vi "az_ellenseg_megtevesztese.vi"() -> ()   [LabVIEW 2018]
uses:
  <vilib>/NI/STM/TCP/TCP Connection Info.ctl
  <vilib>/NI/STM/SubVIs/MetaDataElement.ctl
  <vilib>/NI/STM/TCP/TCP Write Options.ctl
  <vilib>/NI/STM/TCP/TCP Read Options.ctl
  <vilib>/NI/STM/TCP/Write Meta Data (TCP Ref).vi
  <vilib>/NI/STM/TCP/Get Connection Reference (TCP).vi
  <vilib>/NI/STM/TCP/Write Meta Data (TCP Clst).vi
  <vilib>/NI/STM/TCP/Read Message (TCP).vi
  <vilib>/NI/STM/TCP/Write Message (TCP).vi
  <vilib>/NI/STM/NI STM.lvlib
panel:
  out "Sensor not connected":bool
  out "Connected?":bool
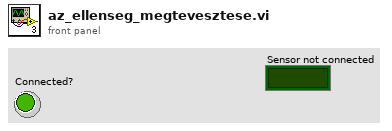
[diagram p1: front panel]
types:
  T1 = typedef "NI STM.lvlib/TCP Connection Info.ctl" = cluster{"connection ID":refnum<k5>, "meta data":T2[]}
  T2 = typedef "NI STM.lvlib/MetaDataElement.ctl" = string
  T3 = typedef "NI STM.lvlib/TCP Write Options.ctl" = cluster{"ignore timeout error":bool, "timeout ms (1000)":i32}
  T4 = typedef "NI STM.lvlib/TCP Read Options.ctl" = cluster{"ignore timeout error":bool, "timeout ms (1000)":i32}
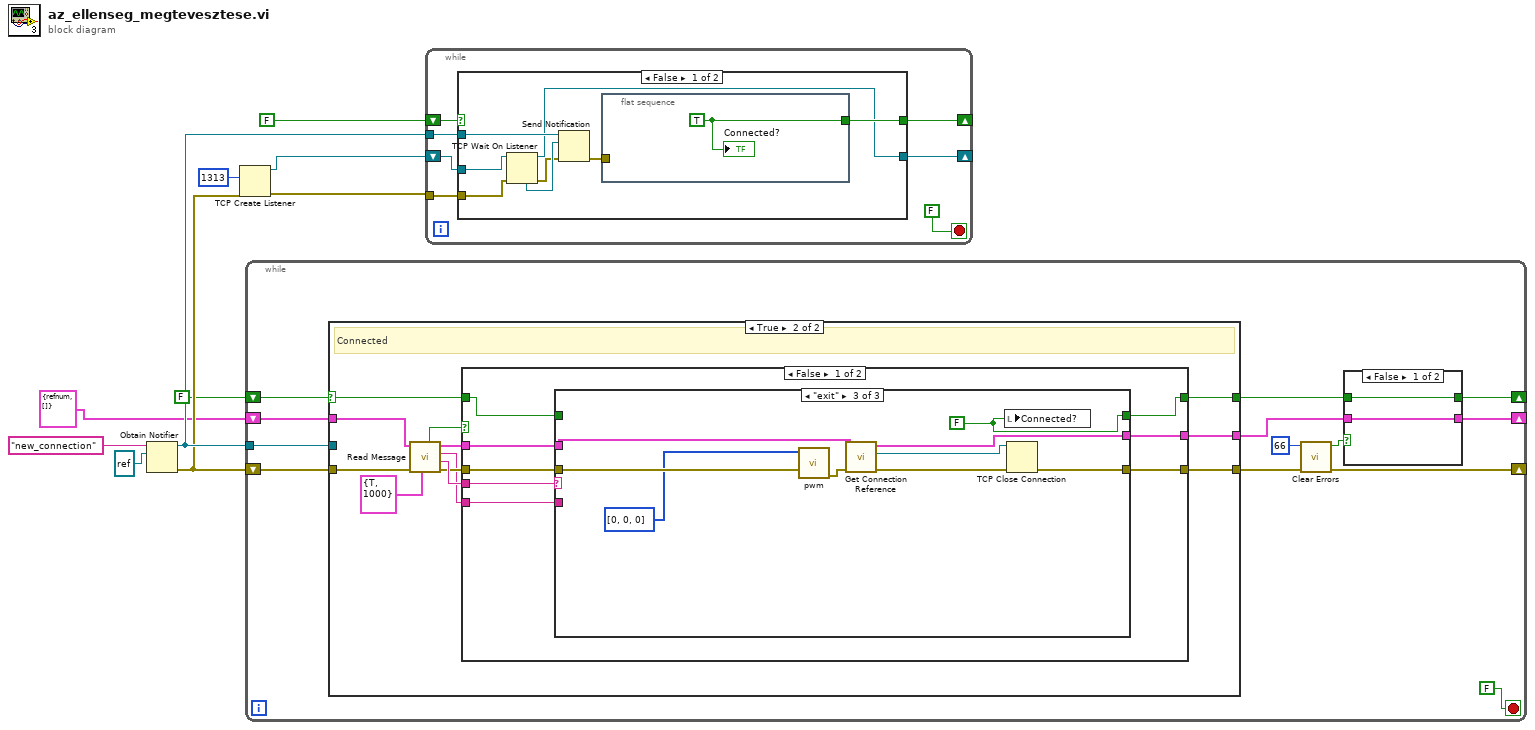
[diagram p0: block diagram]
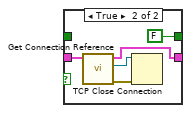
[diagram p2: hidden frame]
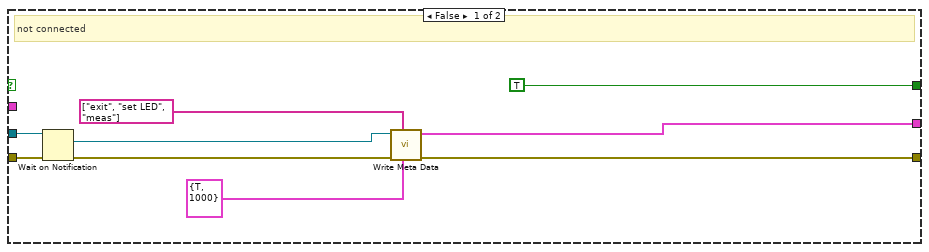
[diagram p3: hidden frame]
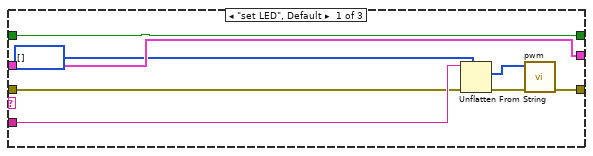
[diagram p4: hidden frame]
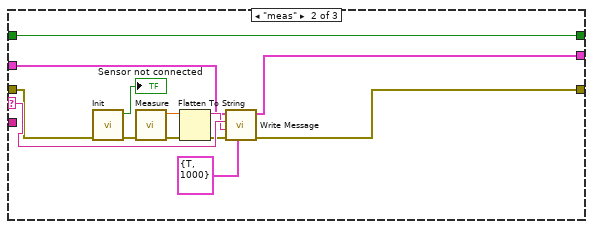
[diagram p5: hidden frame]
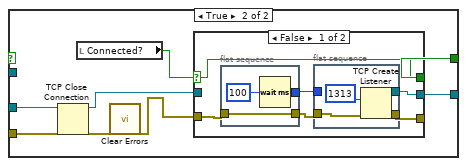
[diagram p7: hidden frame]
diagram:
  n1 = Obtain Notifier(name (unnamed)="new_connection", notification data type=refnum<k5> refnum ("connection ID")) -> (notifier out=w5:refnum<notifier>, error out=w4:errorcluster)  [unwired: 2 in, 1 out]
  n2 = TCP Create Listener(8:w4, 10:u16 1313 ("port")) -> (0:w9:errorcluster, 3:w10:refnum<k5>)  [unwired: 3 in, 1 out]
  n3 = while {
    tunnel: w5 -> [w23]
    shift-right: [w13] -> _
    shift-left: FALSE ("Connected?") -> [w21]
    shift-right: [w11] -> _
    shift-left: T1 {"connection ID"=refnum, "meta data"=[]} ("connection info out") -> [w20]
    shift-right: [w17] -> _
    shift-left: w4 -> [w18]
    stop <- FALSE stop-if-true
    n4 = case shown="True" w21 {
      selector: w21 -> [_ w41]
      tunnel: w23 -> [w39 _]
      tunnel: [TRUE w42] -> w14
      tunnel: [w36 w44] -> w12
      tunnel: w20 -> [_ w50]
      tunnel: [w32 w43] -> w19
      tunnel: w18 -> [w31 w51]
      frame False {
        # "not connected"
        n5 = Wait on Notification(notifier=w39, error in (no error)=w31) -> (notification=w37:refnum<k5>, error out=w35:errorcluster)  [unwired: 2 in, 2 out]
        n6 = call-poly <vilib>:"Write Meta Data.vi"("options"=T3 {"ignore timeout error"=TRUE, "timeout ms (1000)"=1000}, "meta data"=T2[] ["exit", "set LED", "meas"], "error in"=w35, "connection ID"=w37) -> ("error out"=w32:errorcluster, "connection info out"=w36:T1)  [unwired: 6 in]
      }
      frame True {
        # "Connected"
        n7 = call-poly <vilib>:"Read Message.vi"("options"=T4 {"ignore timeout error"=TRUE, "timeout ms (1000)"=1000}, "error in"=w51, "connection info in"=w50) -> ("error out"=w46:errorcluster, "name"=w47:T2, "data string"=w40:string, "connection info out"=w45:T1, "timed out?"=w48:bool)  [unwired: 3 in, 1 out]
        n8 = case shown="False" w48 {
          tunnel: w47 -> [w59 _]
          tunnel: w46 -> [w57 w91]
          tunnel: w45 -> [w58 w92]
          tunnel: [w56 w92] -> w44
          tunnel: [w55 w91] -> w43
          tunnel: [w54 w90] -> w42
          tunnel: w41 -> [w53 w90]
          tunnel: w40 -> [w52 _]
          frame False {
            n9 = case shown="\"exit\"" w59 {
              selector: w59 -> [_ w76 _]
              tunnel: w58 -> [w66 w73 w89]
              tunnel: w57 -> [w61 w70 w83]
              tunnel: [w66 w78 w88] -> w56
              tunnel: [w60 w79 w85] -> w55
              tunnel: [w67 w80 w84] -> w54
              tunnel: w53 -> [w67 w80 _]
              tunnel: w52 -> [w62 _ _]
              frame "set LED", Default {
                n10 = Unflatten From String(type=u8[] [], binary string=w62, error in (no error)=w61) -> (value=w64:u8[], error out=w65:errorcluster)  [unwired: 2 in, 1 out]
                n11 = call "pwm.vi"("Error In"=w65, "PWMs"=w64) -> ("Error Out"=w60:errorcluster)  [unwired: 9 in]
              }
              frame "meas" {
                n12 = call "Init.vi"("Error In"=w70) -> ("Error Out"=w69:errorcluster, "Not connected"=→"Sensor not connected":bool)  [unwired: 9 in]
                n13 = call "Measure.vi"("Error In"=w69) -> ("Error Out"=w72:errorcluster, "Luminosity"=w71:dbl)  [unwired: 9 in]
                n14 = Flatten To String(anything=w71, error in (no error)=w72) -> (data string=w74:string, error out=w75:errorcluster)  [unwired: 2 in, 1 out]
                n15 = call-poly <vilib>:"Write Message.vi"("options"=T3 {"ignore timeout error"=TRUE, "timeout ms (1000)"=1000}, "error in"=w75, "data"=w74, "name"=w76, "connection info in"=w73) -> ("error out"=w79:errorcluster, "connection info out"=w78:T1)  [unwired: 5 in]
              }
              frame "exit" {
                w84 = FALSE ("Connected?")
                n16 = call "pwm.vi"("Error In"=w83, "PWMs"=u8[] [0, 0, 0]) -> ("Error Out"=w82:errorcluster)  [unwired: 9 in]
                n17 = call-poly <vilib>:"Get Connection Reference.vi"("error in"=w82, "connection info in"=w89) -> ("error out"=w87:errorcluster, "connection ID out"=w86:refnum<k5>, "connection info out"=w88:T1)  [unwired: 7 in]
                n18 = local write "Connected?"(w84) -> ()
                n19 = TCP Close Connection(connection ID=w86, error in (no error)=w87) -> (error out=w85:errorcluster)  [unwired: 1 in, 1 out]
              }
            }
          }
          frame True {
          }
        }
      }
    }
    n20 = call <vilib>:"Clear Errors.vi"("error in (no error)"=w19, "specific error code to clear (0: all)"=66) -> ("error out"=w17:errorcluster, "specific error cleared?"=w15:bool)  [unwired: 4 in]
    n21 = case shown="False" w15 {
      tunnel: w14 -> [w25 _]
      tunnel: [w25 FALSE] -> w13
      tunnel: w12 -> [w24 w27]
      tunnel: [w24 w26] -> w11
      frame False {
      }
      frame True {
        n22 = call-poly <vilib>:"Get Connection Reference.vi"("connection info in"=w27) -> ("error out"=w29:errorcluster, "connection ID out"=w30:refnum<k5>, "connection info out"=w26:T1)  [unwired: 8 in]
        n23 = TCP Close Connection(connection ID=w30, error in (no error)=w29) -> ()  [unwired: 1 in, 2 out]
      }
    }
  }
  n24 = while {
    tunnel: w9 -> [w97]
    tunnel: w5 -> [w96]
    shift-right: [w95] -> _
    shift-left: FALSE ("Connected?") -> [w94]
    shift-right: [w93] -> _
    shift-left: w10 -> [w98]
    stop <- FALSE stop-if-true
    n25 = case shown="False" w94 {
      tunnel: w98 -> [w107 w115]
      tunnel: w97 -> [w106 w116]
      tunnel: w96 -> [w105 _]
      tunnel: [w101 w112] -> w95
      tunnel: [w100 w110] -> w93
      frame False {
        n26 = TCP Wait On Listener(8:w106, 11:w107) -> (0:w103:errorcluster, 3:w100:refnum<k5>, 4:w104:refnum<k5>)  [unwired: 2 in, 2 out]
        n27 = Send Notification(notification=w104, notifier=w105, error in (no error)=w103) -> (error out=w102:errorcluster)  [unwired: 1 out]
        n28 = flat-sequence {
          tunnel: w102 -> [_]
          tunnel: [w108] -> w101
          frame #0 {
            w108 = TRUE ("Connected?")
            "Connected?" <- w108
          }
        }
      }
      frame True {
        n29 = TCP Close Connection(connection ID=w115, error in (no error)=w116) -> (connection ID out=w109:refnum<k5>, error out=w114:errorcluster)  [unwired: 1 in]
        n30 = local read "Connected?"() -> (w113:bool)
        n31 = call <vilib>:"Clear Errors.vi"("error in (no error)"=w114) -> ("error out"=w111:errorcluster)  [unwired: 5 in, 1 out]
        n32 = case shown="False" w113 {
          selector: w113 -> [w122 w132]
          tunnel: [w122 w132] -> w112
          tunnel: w111 -> [w118 w130]
          tunnel: [w121 w131] -> w110
          tunnel: w109 -> [_ w131]
          tunnel: [w120 w130] -> _
          frame False {
            n33 = flat-sequence {
              tunnel: [w128] -> w119
              tunnel: w118 -> [w127]
              tunnel: [w127] -> w117
              frame #0 {
                n34 = Wait (ms)(milliseconds to wait=u32 100) -> (millisecond timer value=w128:u32)
              }
            }
            n35 = flat-sequence {
              tunnel: w117 -> [w125]
              tunnel: [w124] -> w121
              tunnel: [w123] -> w120
              tunnel: w119 -> [_]
              frame #0 {
                n36 = TCP Create Listener(8:w125, 10:u16 1313 ("port")) -> (0:w123:errorcluster, 3:w124:refnum<k5>)  [unwired: 3 in, 1 out]
              }
            }
          }
          frame True {
          }
        }
      }
    }
  }
